vi "Get Connected Devices.vi"() -> (3 "List of Device Names to check against what you expect":string[](array[string]))   [LabVIEW 2018]
uses:
  Get Devices JSON.ctl
  <vilib>/httpClient/LabVIEWHTTPClient.lvlib
panel:
  out "JSON converted to LV Cluster":T1
  out "error out":errorcluster
  out "headers":string
  out "body":string
  # "Example Response I got from running \"getversion\""
  # "HTTP/1.1 200 OK\nConnection: keep-alive\nContent-Type: application/json\nContent-Length: 296\nCache-Control: no-cache, no-store"
  # "{\n    \"GeneralReturn\": {\n        \"Action\": \"getversion\",\n        \"Error\": 0,\n        \"ErrorMessage\": \"CTRE_DI_OKAY\",\n        \"ID\": 0,\n        \"Model\": \"\"\n    },\n    \"ReleaseInfo\": \"Kickoff Release\",\n    \"SearchDirectory\": \"/var/volatile/tmp/ctre/\",\n    \"Version\": \"1.0.0 (Jan  1 2019,21:19:48)\"\n}"
  # "Example Response I got from running \"getdevices\""
  # "HTTP/1.1 200 OK\nConnection: keep-alive\nContent-Type: application/json\nContent-Length: 2823\nCache-Control: no-cache, no-store"
  # "{\n    \"DeviceArray\": [\n        {\n            \"BootloaderRev\": \"1.0\",\n            \"CurrentVers\": \"4.13\",\n            \"DynID\": 33878026,\n            \"HardwareRev\": \"1.1\",\n            \"ID\": 33879042,\n            \"ManDate\": \"Nov 9, 2016\",\n            \"Model\": \"Pigeon Over Ribbon\",\n            \"Name\": \"Pigeon connected to Talon SRX (Device ID 2)\",\n            \"SoftStatus\": \"Running Application.\",\n            \"UniqID\": 6,\n            \"Vendor\": \"Cross The Road Electronics\"\n        },\n        {\n            \"BootloaderRev\": \"3.2\",\n            \"CurrentVers\": \"4.11\",\n            \"DynID\": 33880073,\n            \"HardwareRev\": \"1.7\",\n            \"ID\": 33881088,\n            \"ManDate\": \"Aug 14, 2015\",\n            \"Model\": \"Talon SRX\",\n            \"Name\": \"Right Front (Device ID 0)\",\n            \"SoftStatus\": \"Running Application.\",\n            \"UniqID\": 5,\n            \"Vendor\": \"Cross The Road Electronics\"\n        },\n        {\n            \"BootloaderRev\": \"3.2\",\n            \"CurrentVers\": \"4.11\",\n            \"DynID\": 33880071,\n            \"HardwareRev\": \"1.7\",\n            \"ID\": 33881089,\n            \"ManDate\": \"Aug 14, 2015\",\n            \"Model\": \"Talon SRX\",\n            \"Name\": \"Right Back (Device ID 1)\",\n            \"SoftStatus\": \"Running Application.\",\n            \"UniqID\": 3,\n            \"Vendor\": \"Cross The Road Electronics\"\n        },\n        {\n            \"BootloaderRev\": \"3.2\",\n            \"CurrentVers\": \"4.11\",\n            \"DynID\": 33880074,\n            \"HardwareRev\": \"1.7\",\n            \"ID\": 33881090,\n            \"ManDate\": \"Aug 14, 2015\",\n            \"Model\": \"Talon SRX\",\n            \"Name\": \"Left Back (Device ID 2)\",\n            \"SoftStatus\": \"Running Application.\",\n            \"UniqID\": 4,\n            \"Vendor\": \"Cross The Road Electronics\"\n        },\n        {\n            \"BootloaderRev\": \"3.2\",\n            \"CurrentVers\": \"4.11\",\n            \"DynID\": 33880072,\n            \"HardwareRev\": \"1.7\",\n            \"ID\": 33881091,\n            \"ManDate\": \"Aug 14, 2015\",\n            \"Model\": \"Talon SRX\",\n            \"Name\": \"Left Front (Device ID 3)\",\n            \"SoftStatus\": \"Running Application.\",\n            \"UniqID\": 2,\n            \"Vendor\": \"Cross The Road Electronics\"\n        },\n        {\n            \"BootloaderRev\": \"3.1\",\n            \"CurrentVers\": \"1.40\",\n            \"DynID\": 134543366,\n            \"HardwareRev\": \"Smart Module 1.1, Baseboard 1.3\",\n            \"ID\": 134544384,\n            \"ManDate\": \"Nov 4, 2014\",\n            \"Model\": \"PDP\",\n            \"Name\": \"PDP (Device ID 0)\",\n            \"SoftStatus\": \"Running Application.\",\n            \"UniqID\": 7,\n            \"Vendor\": \"Cross The Road Electronics\"\n        }\n    ],\n    \"GeneralReturn\": {\n        \"Action\": \"getdevices\",\n        \"Error\": 0,\n        \"ErrorMessage\": \"CTRE_DI_OKAY\",\n        \"ID\": 0,\n        \"Model\": \"\"\n    }\n}"
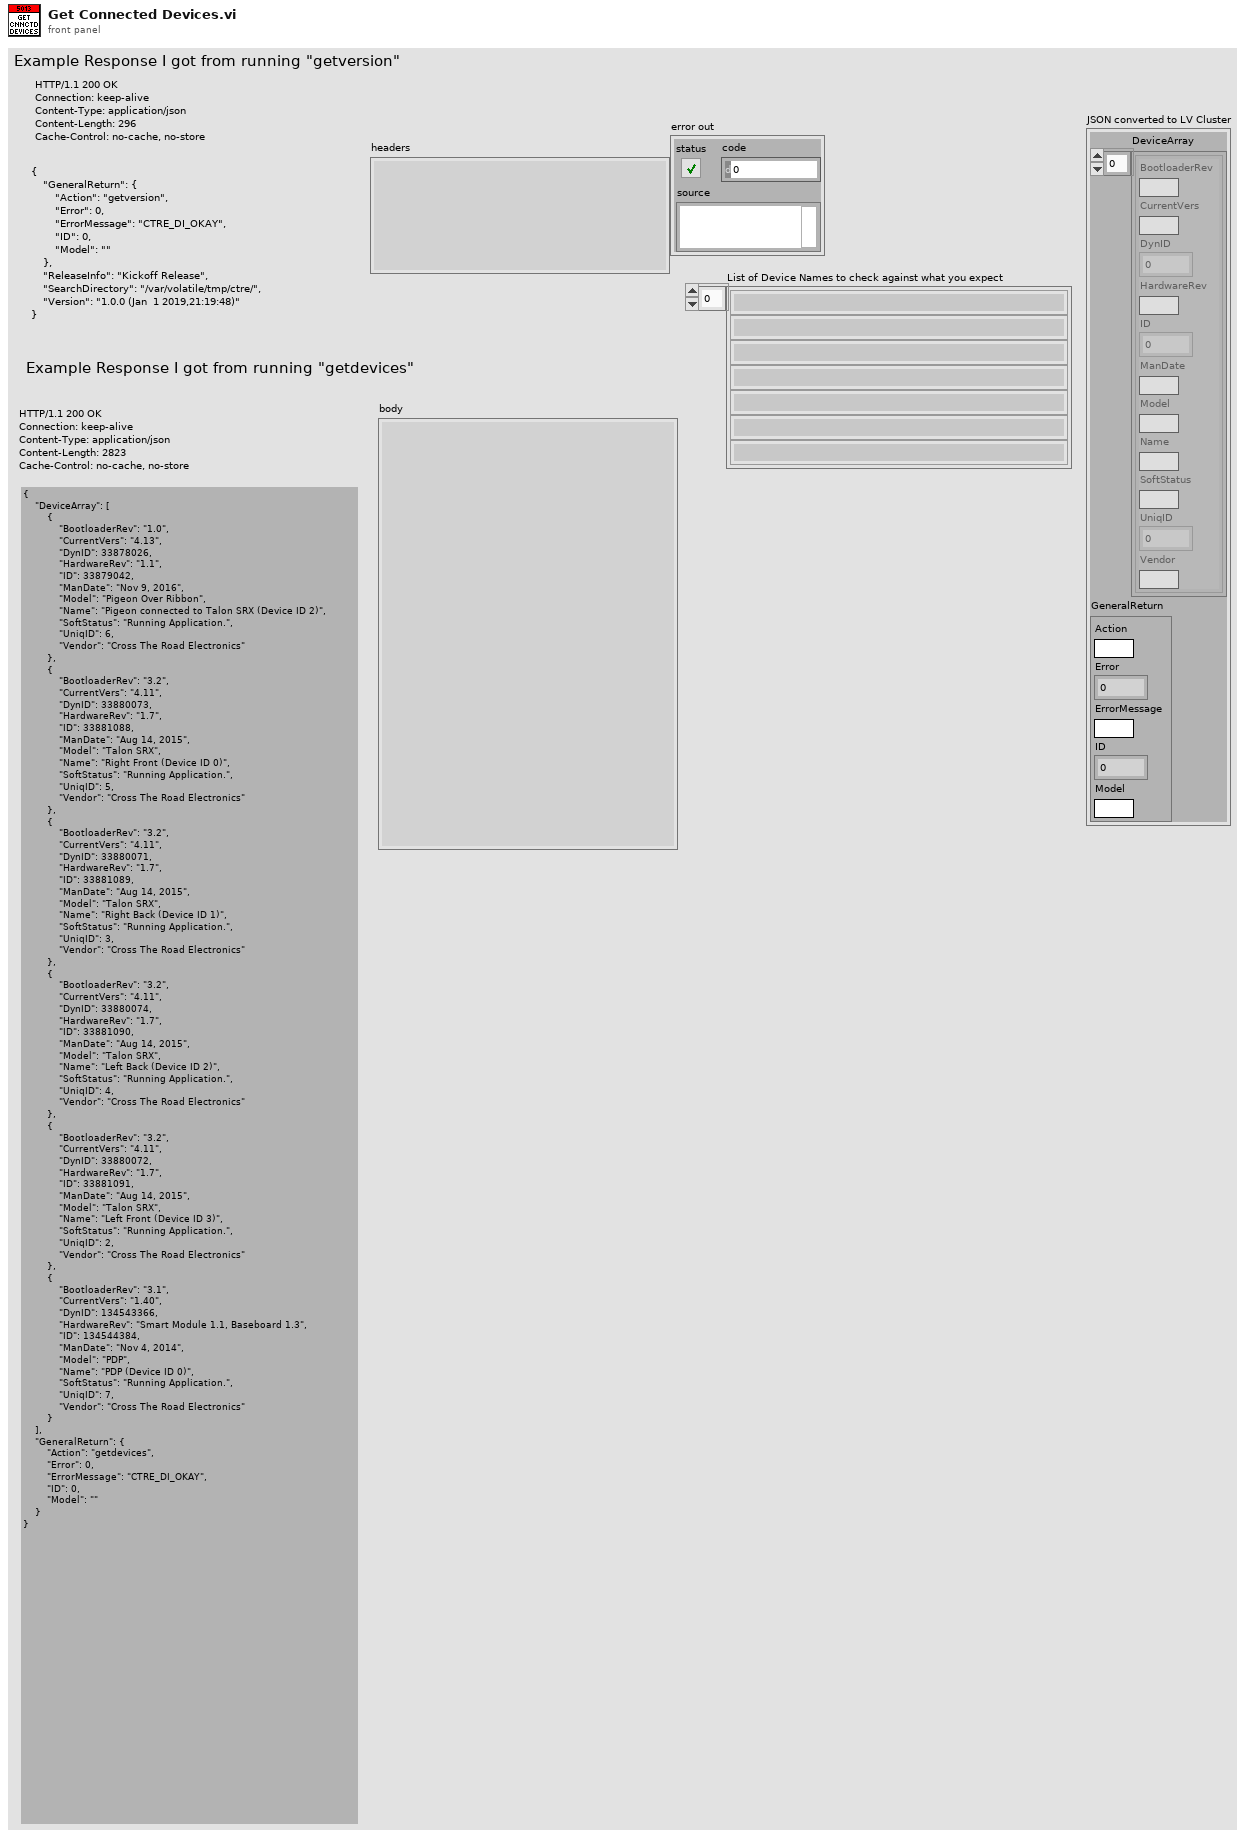
[diagram p1: front panel]
types:
  T1 = typedef "Get Devices JSON.ctl" = cluster{"DeviceArray":cluster{"BootloaderRev":string, "CurrentVers":string, "DynID":dbl, "HardwareRev":string, "ID":dbl, "ManDate":string, "Model":string, "Name":string, "SoftStatus":string, "UniqID":dbl, "Vendor":string}[], "GeneralReturn":cluster{"Action":string, "Error":dbl, "ErrorMessage":string, "ID":dbl, "Model":string}}
  T2 = cluster{"BootloaderRev":string, "CurrentVers":string, "DynID":dbl, "HardwareRev":string, "ID":dbl, "ManDate":string, "Model":string, "Name":string, "SoftStatus":string, "UniqID":dbl, "Vendor":string}[]
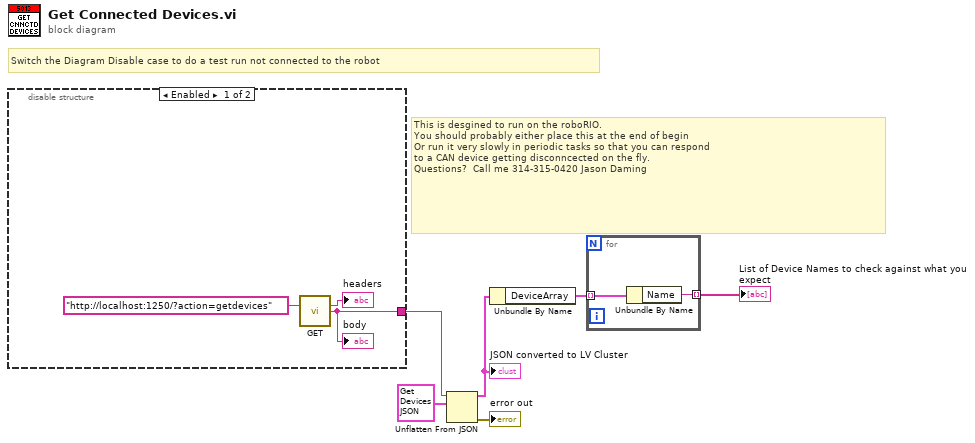
[diagram p0: block diagram]
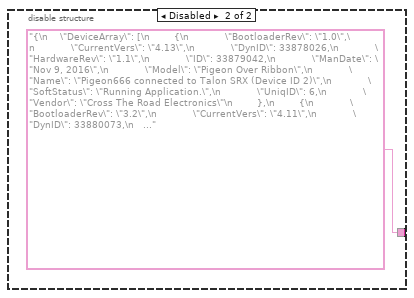
[diagram p2: hidden frame]
diagram:
  # "This is desgined to run on the roboRIO.\nYou should probably either place this at the end of begin\nOr run it very slowly in periodic tasks so that you can respond\nto a CAN device getting disconncected on the fly.\nQuestions?  Call me 314-315-0420 Jason Daming"
  # "Switch the Diagram Disable case to do a test run not connected to the robot"
  n1 = disable-structure shown="Enabled" {
    disable-tunnel: [w7 "{\n    \"DeviceArray\": [\n        {\n            \"BootloaderRev\": \"1.0\",\n            \"CurrentVers\": \"4.13\",\n            \"DynID\": 33878026,\n            \"HardwareRev\": \"1.1\",\n            \"ID\": 33879042,\n            \"ManDate\": \"Nov 9, 2016\",\n            \"Model\": \"Pigeon Over Ribbon\",\n            \"Name\": \"Pigeon666 connected to Talon SRX (Device ID 2)\",\n            \"SoftStatus\": \"Running Application.\",\n            \"UniqID\": 6,\n            \"Vendor\": \"Cross The Road Electronics\"\n        },\n        {\n            \"BootloaderRev\": \"3.2\",\n            \"CurrentVers\": \"4.11\",\n            \"DynID\": 33880073,\n            \"HardwareRev\": \"1.7\",\n            \"ID\": 33881088,\n            \"ManDate\": \"Aug 14, 2015\",\n            \"Model\": \"Talon SRX\",\n            \"Name\": \"Right Front (Device ID 0)\",\n            \"SoftStatus\": \"Running Application.\",\n            \"UniqID\": 5,\n            \"Vendor\": \"Cross The Road Electronics\"\n        },\n        {\n            \"BootloaderRev\": \"3.2\",\n            \"CurrentVers\": \"4.11\",\n            \"DynID\": 33880071,\n            \"HardwareRev\": \"1.7\",\n            \"ID\": 33881089,\n            \"ManDate\": \"Aug 14, 2015\",\n            \"Model\": \"Talon SRX\",\n            \"Name\": \"Right Back (Device ID 1)\",\n            \"SoftStatus\": \"Running Application.\",\n            \"UniqID\": 3,\n            \"Vendor\": \"Cross The Road Electronics\"\n        },\n        {\n            \"BootloaderRev\": \"3.2\",\n            \"CurrentVers\": \"4.11\",\n            \"DynID\": 33880074,\n            \"HardwareRev\": \"1.7\",\n            \"ID\": 33881090,\n            \"ManDate\": \"Aug 14, 2015\",\n            \"Model\": \"Talon SRX\",\n            \"Name\": \"Left Back (Device ID 2)\",\n            \"SoftStatus\": \"Running Application.\",\n            \"UniqID\": 4,\n            \"Vendor\": \"Cross The Road Electronics\"\n        },\n        {\n            \"BootloaderRev\": \"3.2\",\n            \"CurrentVers\": \"4.11\",\n            \"DynID\": 33880072,\n            \"HardwareRev\": \"1.7\",\n            \"ID\": 33881091,\n            \"ManDate\": \"Aug 14, 2015\",\n            \"Model\": \"Talon SRX\",\n            \"Name\": \"Left Front (Device ID 3)\",\n            \"SoftStatus\": \"Running Application.\",\n            \"UniqID\": 2,\n            \"Vendor\": \"Cross The Road Electronics\"\n        },\n        {\n            \"BootloaderRev\": \"3.1\",\n            \"CurrentVers\": \"1.40\",\n            \"DynID\": 134543366,\n            \"HardwareRev\": \"Smart Module 1.1, Baseboard 1.3\",\n            \"ID\": 134544384,\n            \"ManDate\": \"Nov 4, 2014\",\n            \"Model\": \"PDP\",\n            \"Name\": \"PDP (Device ID 0)\",\n            \"SoftStatus\": \"Running Application.\",\n            \"UniqID\": 7,\n            \"Vendor\": \"Cross The Road Electronics\"\n        }\n    ],\n    \"GeneralReturn\": {\n        \"Action\": \"getdevices\",\n        \"Error\": 0,\n        \"ErrorMessage\": \"CTRE_DI_OKAY\",\n        \"ID\": 0,\n        \"Model\": \"\"\n    }\n}" ("body")] -> w6
    frame Enabled {
      n2 = call <vilib>:"GET.vi"("url"="http://localhost:1250/?action=getdevices") -> ("headers"=→"headers":string, "body"=w7:string)  [unwired: 11 in, 2 out]
      "body" <- w7
    }
    frame Disabled {
    }
  }
  n3 = Unflatten From JSON(JSON string=w6, type and defaults=T1 {"DeviceArray"=[{"BootloaderRev"="1.0", "CurrentVers"="4.13", "DynID"=33878026.0, "HardwareRev"="1.1", "ID"=33879042.0, "ManDate"="Nov 9, 2016", "Model"="Pigeon Over Ribbon", "Name"="Pigeon connected to Talon SRX (Device ID 2)", "SoftStatus"="Running Application.", "UniqID"=6.0, "Vendor"="Cross The Road Electronics"}, {"BootloaderRev"="3.2", "CurrentVers"="4.11", "DynID"=33880073.0, "HardwareRev"="1.7", "ID"=33881088.0, "ManDate"="Aug 14, 2015", "Model"="Talon SRX", "Name"="Right Front (Device ID 0)", "SoftStatus"="Running Application.", "UniqID"=5.0, "Vendor"="Cross The Road Electronics"}, {"BootloaderRev"="3.2", "CurrentVers"="4.11", "DynID"=33880071.0, "HardwareRev"="1.7", "ID"=33881089.0, "ManDate"="Aug 14, 2015", "Model"="Talon SRX", "Name"="Right Back (Device ID 1)", "SoftStatus"="Running Application.", "UniqID"=3.0, "Vendor"="Cross The Road Electronics"}, {"BootloaderRev"="3.2", "CurrentVers"="4.11", "DynID"=33880074.0, "HardwareRev"="1.7", "ID"=33881090.0, "ManDate"="Aug 14, 2015", "Model"="Talon SRX", "Name"="Left Back (Device ID 2)", "SoftStatus"="Running Application.", "UniqID"=4.0, "Vendor"="Cross The Road Electronics"}, {"BootloaderRev"="3.2", "CurrentVers"="4.11", "DynID"=33880072.0, "HardwareRev"="1.7", "ID"=33881091.0, "ManDate"="Aug 14, 2015", "Model"="Talon SRX", "Name"="Left Front (Device ID 3)", "SoftStatus"="Running Application.", "UniqID"=2.0, "Vendor"="Cross The Road Electronics"}, {"BootloaderRev"="3.1", "CurrentVers"="1.40", "DynID"=134543366.0, "HardwareRev"="Smart Module 1.1, Baseboard 1.3", "ID"=134544384.0, "ManDate"="Nov 4, 2014", "Model"="PDP", "Name"="PDP (Device ID 0)", "SoftStatus"="Running Application.", "UniqID"=7.0, "Vendor"="Cross The Road Electronics"}], "GeneralReturn"={"Action"="getdevices", "Error"=0.0, "ErrorMessage"="CTRE_DI_OKAY", "ID"=0.0, "Model"=""}} ("Parsed Data")) -> (value=w3:T1, error out=→"error out":errorcluster)  [unwired: 5 in]
  "JSON converted to LV Cluster" <- w3
  n4 = Unbundle By Name(w3) -> ("DeviceArray"=w2:T2)
  n5 = for {
    tunnel: w2 -> [w12] mode=indexing
    tunnel: [w11] -> w1 mode=indexing
    n6 = Unbundle By Name(w12) -> ("Name"=w11:string)
  }
  "List of Device Names to check against what you expect" <- w1
